vi "protocoljunk1.vi"() -> ()   [LabVIEW 2013]
uses:
  <vilib>/Utility/NIReport.llb/NI_report.lvclass
  General VIs/Tesla/Control/Command Enum.ctl
  <vilib>/Utility/NIReport.llb/Append Report Text (str wrap).vi
panel:
  in  "Panic Stop":bool=TRUE
  out "lengh":i32
  out "size(s)":i32
  out "count":i32
  out "subarray":string[](array[string])
  out "hex integer string":string[](array[string])
  out "error out":errorcluster
  in  "error in":errorcluster
  out "index":i32
  # "t"
  # "=0"
  # "l"
  # "v"
  # "v"
  # "t"
  # "=4"
  # "l"
  # "v"
  # "v"
  # "v"
  # "v"
  # "v"
  # "v"
  # "v"
  # "v"
  # "t"
  # "l"
  # "v"
  # "v"
  # "T"
  # "v"
  # "v"
  # "v"
  # "v"
  # "t"
  # "l"
  # "v"
  # "v"
  # "v"
  # "v"
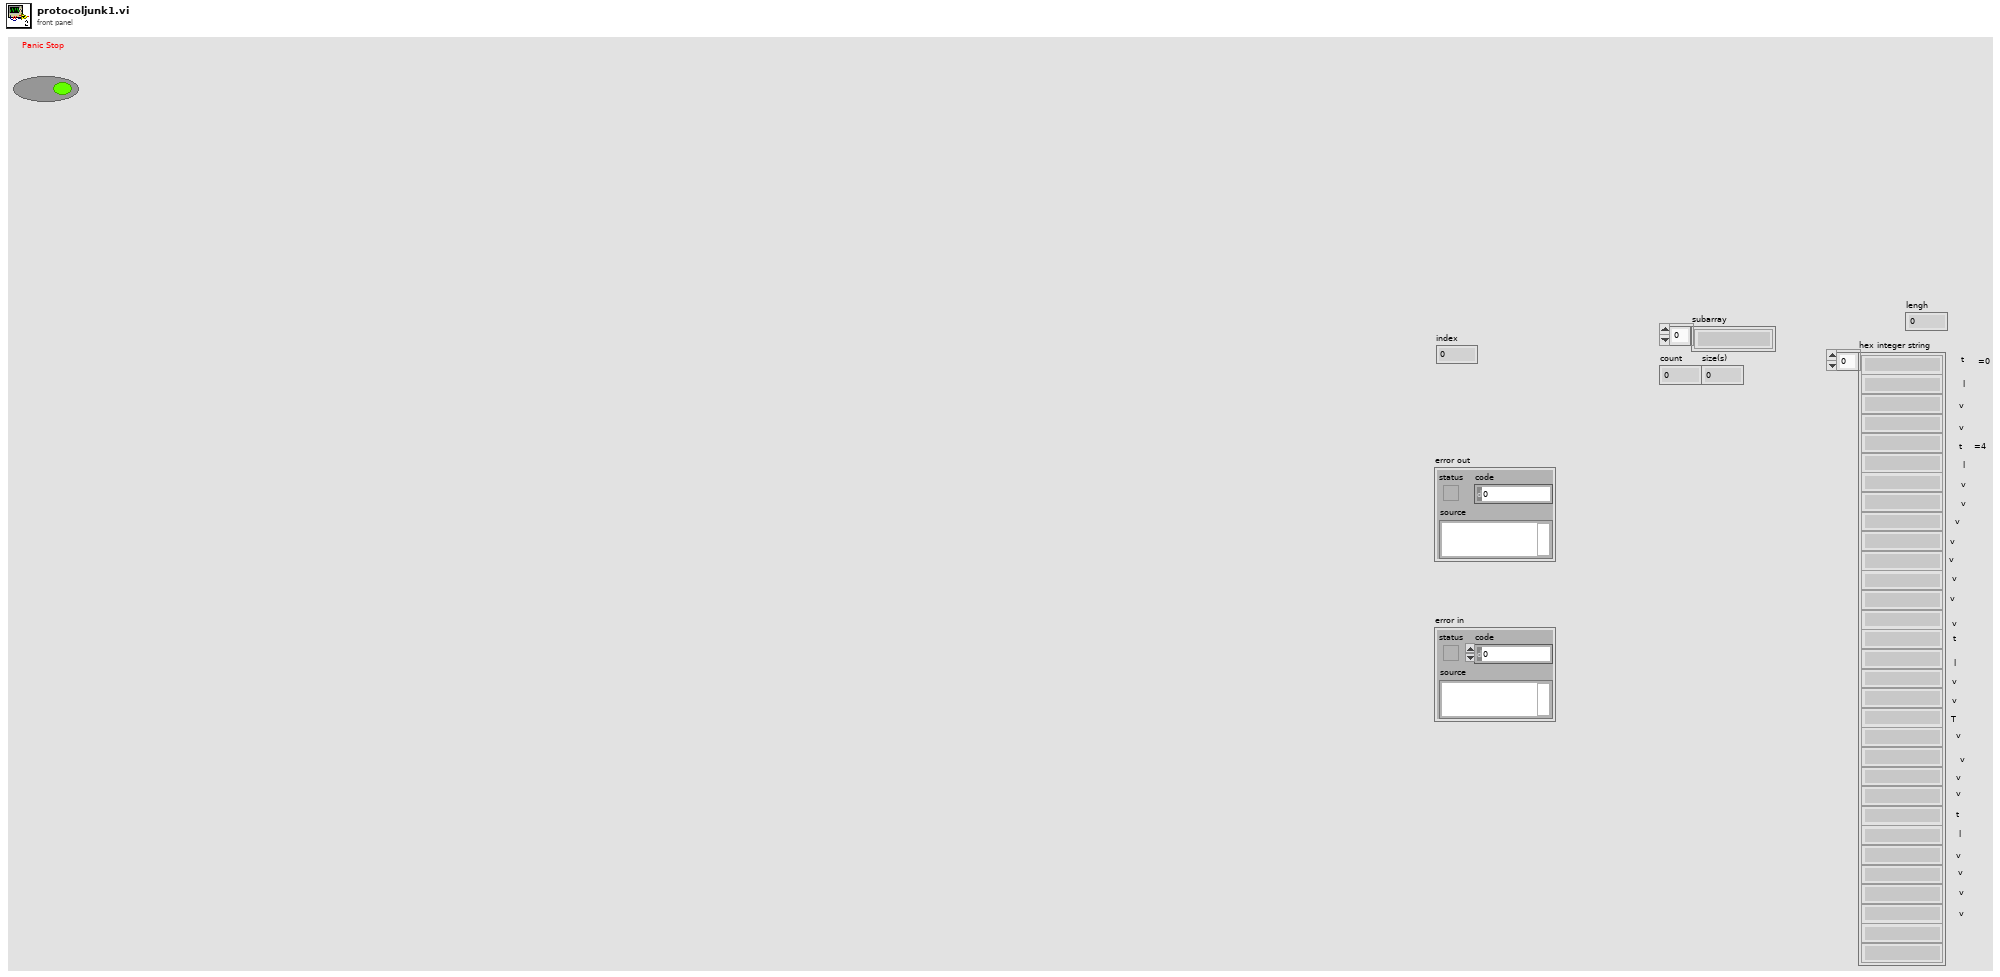
[diagram p1: front panel]
types:
  T1 = cluster{"Charset (-1)":i16, "Weight (-1)":i16, "Name":string, "Size":string}
  T2 = enum16{"Standard Report", "HTML", "Word", "Excel"}
  T3 = enum16{"big-endian, network order", "native, host order", "little-endian"}
  T4 = enum16{"open", "replace", "create", "open or create", "replace or create", "replace or create with confirmation"}
  T5 = typedef "Command Enum.ctl" = enum16{"Test Selection", "Network", "Text Base", "Protocol", "Restart_Print", "Stop"}
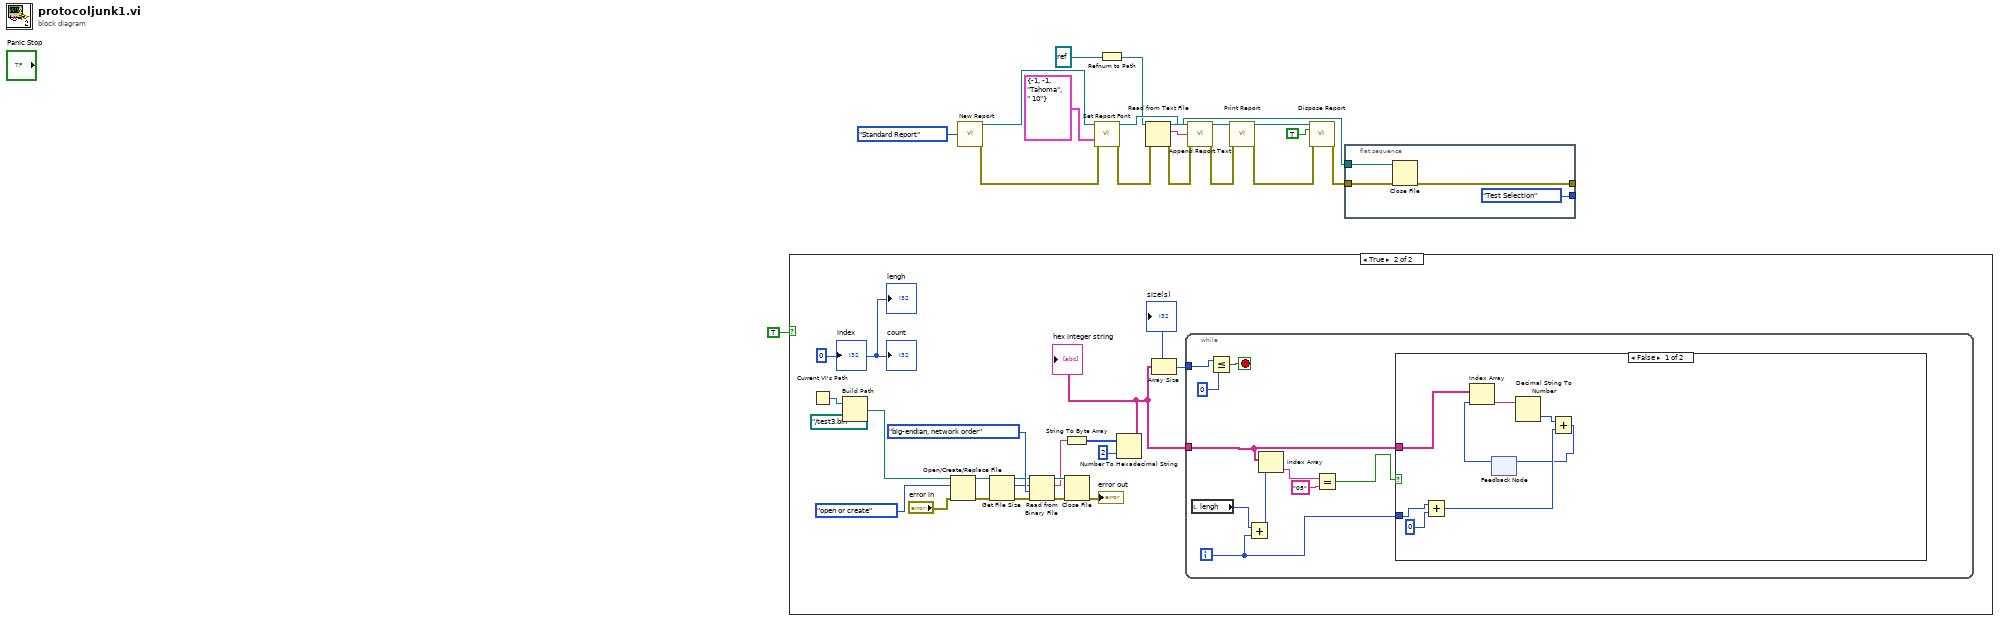
[diagram p0: block diagram]
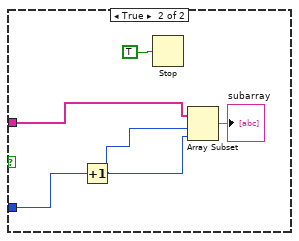
[diagram p3: hidden frame]
diagram:
  n1 = case shown="True" TRUE {
    frame False {
    }
    frame True {
      w19 = 0
      n2 = Current VI's Path() -> (path=w23:path)
      n3 = Build Path(base path=w23, name or relative path=path "../test3.bin") -> (appended path=w22:path)
      n4 = Open/Create/Replace File(file path (use dialog)=w22, error in="error in", operation (0:open)=T4."open or create") -> (refnum out=w32:refnum<file>, error out=w30:errorcluster)  [unwired: 3 in, 1 out]
      n5 = Get File Size(file=w32, error in=w30) -> (refnum out=w31:refnum<file>, size (in bytes)=w28:i64, 0:w29:errorcluster)
      n6 = Read from Binary File(8:w29, 9:T3."big-endian, network order" ("byte order (0:big-endian, network order)"), 10:w28, 11:w31) -> (0:w35:errorcluster, 2:w27:string, 3:w33:refnum<file>)  [unwired: 2 in, 1 out]
      n7 = String To Byte Array(string=w27) -> (unsigned byte array=w26:u8[])
      n8 = Close File(refnum=w33, error in=w35) -> (error out=→"error out":errorcluster)  [unwired: 1 out]
      n9 = Number To Hexadecimal String(1:2, 2:w26) -> (0:w24:string[])
      "hex integer string" <- w24
      n10 = Array Size(array=w24) -> (size(s)=w20:i32)
      "size(s)" <- w20
      n11 = while {
        tunnel: w24 -> [w43]
        tunnel: w20 -> [w46]
        i -> [w40]
        stop <- w45 stop-if-true
        n12 = local read "lengh"() -> (w41:i32)
        n13 = Less Or Equal?(x=w46, y=0) -> (x <= y?=w45:bool)
        n14 = Add(x=w41, y=w40) -> (x+y=w39:i32)
        n15 = Index Array(array=w43, index=w39) -> (element=w47:string)
        n16 = Equal?(x=w47, y="05") -> (x = y?=w44:bool)
        n17 = case shown="False" w44 {
          tunnel: w43 -> [w55 w61]
          tunnel: w40 -> [w54 w57]
          frame False {
            n18 = Add(x=w54, y=0) -> (x+y=w51:i32)
            n19 = feedback #1() -> (w49:i32)  [unwired: 1 in]
            n20 = Index Array(array=w55, index=w49) -> (element=w56:string)
            n21 = Decimal String To Number(string=w56) -> (number=w52:i32)  [unwired: 2 in, 1 out]
            n22 = Add(x=w52, y=w51) -> (x+y=w50:i32)
            n23 = feedback-in #1(w50) -> ()
          }
          frame True {
            n24 = Increment(x=w57) -> (x+1=w60:i32)
            n25 = Stop(stop? (T)=TRUE) -> ()
            n26 = Array Subset(array=w61, index=w60, length=w60) -> (→"subarray":string[])
          }
        }
      }
      "index" <- w19
      "count" <- w19
      "lengh" <- w19
    }
  }
  n27 = call <vilib>:"New Report.vi"("report type"=T2."Standard Report") -> ("report out"=w15:refnum<class "NI_report.lvclass">, "error out"=w16:errorcluster)  [unwired: 13 in]
  n28 = call-dynamic "Set Report Font.vi"("report in"=w15, "font settings"=T1 {"Charset (-1)"=-1, "Weight (-1)"=-1, "Name"="Tahoma", "Size"=" 10"}, "error in (no error)"=w16) -> ("report out"=w14:refnum<class "NI_report.lvclass">, "error out"=w13:errorcluster)  [unwired: 10 in, 1 out]
  n29 = Refnum to Path(1:refnum<file> refnum ("refnum")) -> (0:w2:path)
  n30 = Read from Text File(file (use dialog)=w2, error in=w13) -> (refnum out=w3:refnum<file>, text=w12:string, error out=w11:errorcluster)  [unwired: 2 in, 1 out]
  n31 = call-poly <vilib>:"Append Report Text.vi"("report in"=w14, "text"=w12, "error in (no error)"=w11) -> ("report out"=w10:refnum<class "NI_report.lvclass">, "error out"=w7:errorcluster)  [unwired: 9 in, 2 out]
  n32 = call-dynamic "Print Report.vi"("report in"=w10, "error in (no error)"=w7) -> ("report out"=w8:refnum<class "NI_report.lvclass">, "error out"=w9:errorcluster)  [unwired: 12 in]
  n33 = call-dynamic "Dispose Report.vi"("report in"=w8, "wait until printing completed? (T)"=TRUE, "error in (no error)"=w9) -> ("error out"=w4:errorcluster)  [unwired: 12 in]
  n34 = flat-sequence {
    tunnel: w4 -> [w65]
    tunnel: [w64] -> _
    tunnel: w3 -> [w63]
    tunnel: [Command_Enum."Test Selection" ("Command Enum")] -> _
    frame #0 {
      n35 = Close File(refnum=w63, error in=w65) -> (error out=w64:errorcluster)  [unwired: 1 out]
    }
  }
